vi "Spreadsheet Write.vi"(0 "Initial Path":path=path "Z:/", 1 "transpose? (no:F)":bool, 4 "format (%.3f)":string="%.3f", 5 "append to file? (new file:F)":bool, 6 "Header Strings":string[](array[string]), 7 "2D data":sgl[][](array[numeric]) format="%.2f", 8 "file path (dialog if empty)":path) -> (2 "error out":errorcluster={"status"=TRUE, "code"=43, "source"="File Dialog"}, 3 "new file path (Not A Path if cancelled)":path)   [LabVIEW 2019]
doc: "This VI is identical to the standard Write To Spreadsheet File VI except that instead of passing the error cluster to the General Error Handler VI, it makes the error cluster available at a terminal."
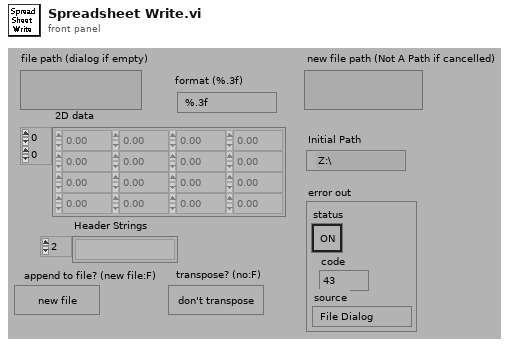
[diagram p1: front panel]
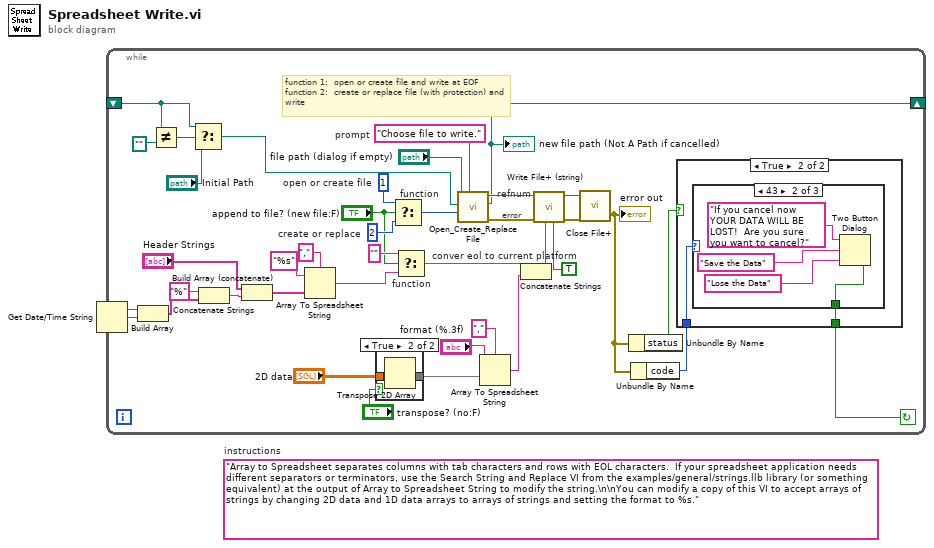
[diagram p0: block diagram]
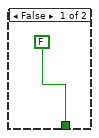
[diagram p2: hidden frame]
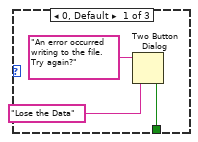
[diagram p3: hidden frame]
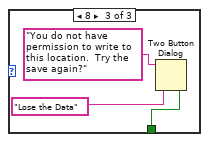
[diagram p4: hidden frame]
diagram:
  (unwired) "Array to Spreadsheet separates columns with tab characters and rows with EOL characters.  If your spreadsheet application needs different separators or terminators, use the Search String and Replace VI from the examples/general/strings.llb library (or something equivalent) at the output of Array to Spreadsheet String to modify the string.\n\nYou can modify a copy of this VI to accept arrays of strings by changing 2D data and 1D data arrays to arrays of strings and setting the format to %s."  # instructions
  n1 = while {
    shift-right: [w11] -> _
    shift-left: _ -> [w7]
    stop <- w24 continue-if-true
    w28 = i16 2  # create or replace
    w30 = TRUE  # conver eol to current platform
    w33 = "Choose file to write."  # prompt
    w40 = i16 1  # open or create file
    # "error"
    # "refnum"
    # "function 1:  open or create file and write at EOF\nfunction 2:  create or replace file (with protection) and write"
    n2 = Get Date/Time String() -> (date string=w15:string, time string=w16:string)  [unwired: 3 in]
    n3 = Build Array(w15, w16) -> (w3:string[])
    n4 = Not Equal?(x=w7, y=path "") -> (x != y?=w9:bool)
    n5 = Select(t=w7, s=w9, f="Initial Path") -> (s? t:f=w6:path)
    n6 = Concatenate Strings("%" ("string"), w3) -> (w4:string)
    n7 = Build Array (concatenate)("Header Strings", w4) -> (w12:string[])
    n8 = Array To Spreadsheet String(delimiter (Tab)=",", array=w12, 3:"%s" ("format string")) -> (spreadsheet string=w13:string)
    n9 = case shown="True" "transpose? (no:F)" {
      tunnel: [w54 w56] -> w36
      tunnel: "2D data" -> [w54 w55]
      frame False {
      }
      frame True {
        n10 = Transpose 2D Array(2D array=w55) -> (transposed array=w56:sgl[][])
      }
    }
    n11 = Select "function"(t=w40, s="append to file? (new file:F)", f=w28) -> (s? t:f=w35:i16)
    n12 = Select "function"(t="", s="append to file? (new file:F)", f=w13) -> (s? t:f=w22:string)
    n13 = call <vilib>:"Open_Create_Replace File.vi"("prompt"=w33, "function (open:0)"=w35, "start path  (Not A Path)"=w6, "file path"="file path (dialog if empty)") -> ("error out"=w32:errorcluster, "new file path"=w11:path, "refnum"=w29:refnum<file>)  [unwired: 4 in, 1 out]
    "new file path (Not A Path if cancelled)" <- w11
    n14 = Array To Spreadsheet String(delimiter (Tab)=",", array=w36, 3:"format (%.3f)") -> (spreadsheet string=w25:string)
    n15 = Concatenate Strings(w22, w25) -> (w26:string)
    n16 = call <vilib>:"Write File+ (string).vi"("convert eol? (no:F)"=w30, "string"=w26, "error in (no error)"=w32, "refnum"=w29) -> ("error out"=w39:errorcluster, "dup refnum"=w31:refnum<file>)  [unwired: 3 in, 1 out]
    n17 = call <vilib>:"Close File+.vi"("error in (no error)"=w39, "refnum"=w31) -> ("error out"=w23:errorcluster)  [unwired: 3 in, 2 out]
    "error out" <- w23
    n18 = Unbundle By Name(w23) -> ("status"=w19:bool)
    n19 = Unbundle By Name(w23) -> ("code"=w18:i32)
    n20 = case shown="True" w19 {
      tunnel: [FALSE ("T button?") w43] -> w24
      tunnel: w18 -> [_ w42]
      frame False {
      }
      frame True {
        n21 = case shown="43" w42 {
          tunnel: [w45 w47 w52] -> w43
          frame 0, Default {
            n22 = Two Button Dialog(message="An error occurred writing to the file.  Try again?", 1:"Lose the Data" ("F button name (\"Cancel\")")) -> (T button?=w45:bool)  [unwired: 1 in]
          }
          frame 43 {
            n23 = Two Button Dialog(message="If you cancel now YOUR DATA WILL BE LOST!  Are you sure you want to cancel?", 1:"Lose the Data" ("F button name (\"Cancel\")"), 2:"Save the Data" ("T button name (\"OK\")")) -> (T button?=w47:bool)
          }
          frame 8 {
            n24 = Two Button Dialog(message="You do not have permission to write to this location.  Try the save again?", 1:"Lose the Data" ("F button name (\"Cancel\")")) -> (T button?=w52:bool)  [unwired: 1 in]
          }
        }
      }
    }
  }
